vi "Implement Motor Voltage Outputs.vi"   [LabVIEW 2009]
uses:
  <vilib>/eio/EIONode/EIONode.xnode
  Motor Encoder Global.vi
  Motor Output Global.vi
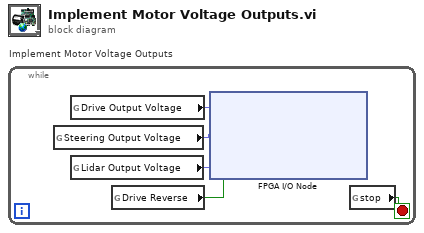
[diagram p0: block diagram]
diagram:
  n1 = while "Implement Motor Voltage Outputs" {
    stop <- w1 stop-if-true
    n2 = global read "Motor Output Global.vi" "Steering Output Voltage"() -> (w3:fxp<+/-,20,5>)
    n3 = global read "Motor Output Global.vi" "Drive Output Voltage"() -> (w5:fxp<+/-,20,5>)
    n4 = global read "Motor Output Global.vi" "Lidar Output Voltage"() -> (w4:fxp<+/-,20,5>)
    n5 = global read "Motor Output Global.vi" "Drive Reverse"() -> (w2:bool)
    n6 = xnode "FPGA I/O Node"("Drive Motor Speed"=w5, "Steering Motor Speed"=w3, "Lidar Motor Speed"=w4, "Drive Motor Reverse"=w2) -> ()  [unwired: 4 in, 4 out]
    n7 = global read "Motor Encoder Global.vi" "stop"() -> (w1:bool)
  }
